vi "Entry.vi"(8 "error in (no error)":errorcluster, 11 "Automation Controller in":refnum<class "Automation Controller.lvclass">) -> (0 "error out":errorcluster, 3 "Automation Controller out":refnum<class "Automation Controller.lvclass">)   [LabVIEW 2024]
uses:
  Automation Controller.lvclass/Automation Controller.ctl
  Automation Controller.lvclass
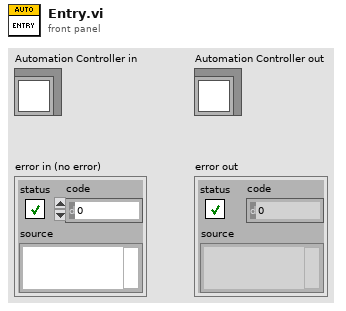
[diagram p1: front panel]
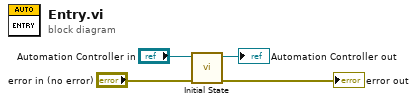
[diagram p0: block diagram]
diagram:
  n1 = call "Initial State.vi"("error in (no error)"="error in (no error)", "Automation Controller in"="Automation Controller in") -> ("error out"=→"error out":errorcluster, "Automation Controller out"=→"Automation Controller out":refnum<class "Automation Controller.lvclass">)  [unwired: 8 in]
